vi "TDTSyn-Get CAR Channel Counts.vi"(0 "Synapse URL":string, 11 "error in (no error)":errorcluster) -> (4 "Channel counts":i32[](array[numeric]), 15 "error out":errorcluster)   [LabVIEW 2020]
uses:
  <vilib>/regexp/Match Regular Expression.xnode
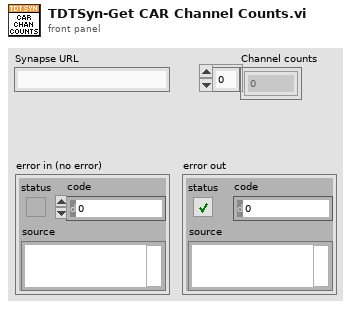
[diagram p1: front panel]
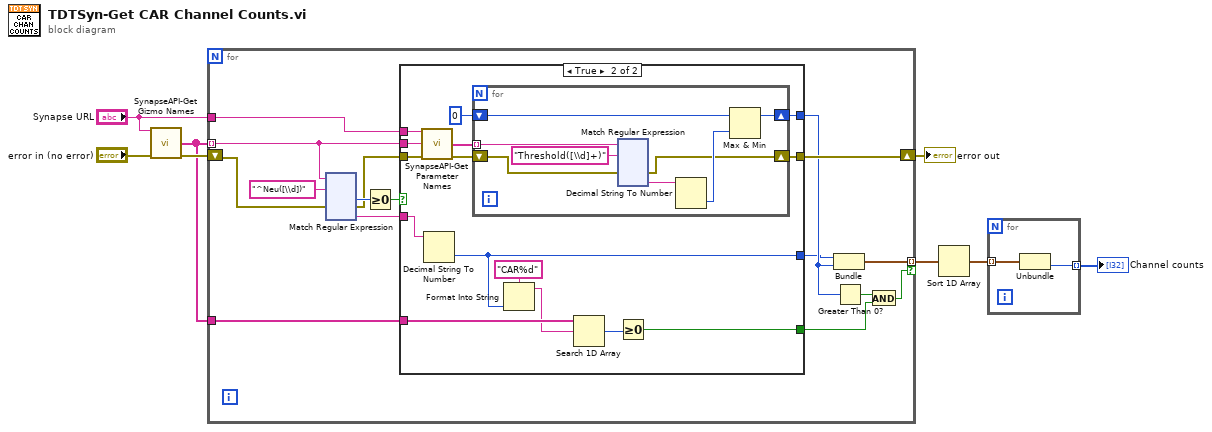
[diagram p0: block diagram]
diagram:
  n1 = call "SynapseAPI-Get Gizmo Names.vi"("URL"="Synapse URL", "error in (no error)"="error in (no error)") -> ("names"=w4:string[], "error out"=w7:errorcluster)  [unwired: 12 in]
  n2 = for {
    tunnel: w4 -> [w19] mode=indexing
    shift-right: [w18] -> w5
    shift-left: w7 -> [w23]
    tunnel: "Synapse URL" -> [w24]
    tunnel: [w14] -> w3 mode=indexing if=w9
    tunnel: w4 -> [w12]
    n3 = xnode "Match Regular Expression"("input string"=w19, "regular expression"="^Neu([\\d])", "error in"=w23) -> ("offset past match"=w22:i32, "error out"=w21:errorcluster, "submatch 1"=w15:string)  [unwired: 3 in, 3 out]
    n4 = Greater Or Equal To 0?(x=w22) -> (x >= 0?=w20:bool)
    n5 = case shown="True" w20 {
      tunnel: w24 -> [_ w40]
      tunnel: w21 -> [w25 w39]
      tunnel: w19 -> [_ w38]
      tunnel: [_ w34] -> w17
      tunnel: [w25 w33] -> w18
      tunnel: w15 -> [_ w32]
      tunnel: [_ w30] -> w13
      tunnel: w12 -> [_ w29]
      tunnel: [_ w26] -> w10
      frame False {
      }
      frame True {
        n6 = call "SynapseAPI-Get Parameter Names.vi"("URL"=w40, "gizmo"=w38, "error in (no error)"=w39) -> ("parameters"=w36:string[], "error out"=w37:errorcluster)  [unwired: 11 in]
        n7 = Decimal String To Number(string=w32) -> (number=w30:i32)  [unwired: 2 in, 1 out]
        n8 = for {
          shift-right: [w42] -> w33
          shift-left: w37 -> [w47]
          tunnel: w36 -> [w48] mode=indexing
          shift-right: [w45] -> w34
          shift-left: 0 -> [w44]
          n9 = xnode "Match Regular Expression"("input string"=w48, "regular expression"="Threshold([\\d]+)", "error in"=w47) -> ("error out"=w42:errorcluster, "submatch 1"=w41:string)  [unwired: 3 in, 4 out]
          n10 = Decimal String To Number(string=w41) -> (number=w43:i32)  [unwired: 2 in, 1 out]
          n11 = Max & Min(x=w44, y=w43) -> (max(x,y)=w45:i32)  [unwired: 1 out]
        }
        n12 = Format Into String(format string="CAR%d", w30) -> (resulting string=w28:string)  [unwired: 2 in, 1 out]
        n13 = Search 1D Array(1D array=w29, element=w28) -> (index of element=w27:i32)  [unwired: 1 in]
        n14 = Greater Or Equal To 0?(x=w27) -> (x >= 0?=w26:bool)
      }
    }
    n15 = Bundle(w13, w17) -> (w14:cluster{i32, i32})  [unwired: 1 in]
    n16 = Greater Than 0?(x=w17) -> (x > 0?=w11:bool)
    n17 = And(x=w11, y=w10) -> (x .and. y?=w9:bool)
  }
  "error out" <- w5
  n18 = Sort 1D Array(array=w3) -> (sorted array=w2:cluster{i32, i32}[])
  n19 = for {
    tunnel: w2 -> [w282] mode=indexing
    tunnel: [w281] -> w1 mode=indexing
    n20 = Unbundle(w282) -> (w281:i32)  [unwired: 1 out]
  }
  "Channel counts" <- w1
